vi "Magnetic_Force.vi"() -> ()   [LabVIEW 2022 SP3]
panel:
  out "Force (N/m)":dbl
  in  "Distance (m)":dbl
  in  "Current 2 (A)":dbl
  in  "Current 1 (A)":dbl
  # "Magnetic_Force:\n2 wires carrying a current will enact a \nmagnetic force upon each other. This force\nper unit length of wire will be calculated given\ninputs of current in each wire and the distance\nbetween said wires."
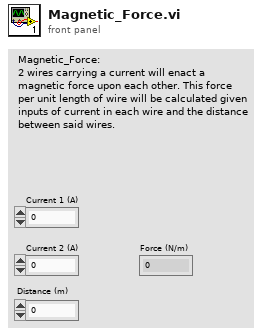
[diagram p1: front panel]
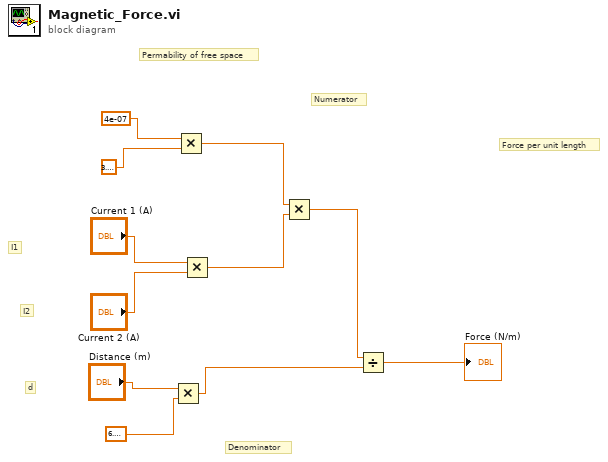
[diagram p0: block diagram]
diagram:
  # "Force per unit length"
  # "Denominator"
  # "Numerator"
  # "d"
  # "I2"
  # "I1"
  # "Permability of free space"
  n1 = Multiply(x="Distance (m)", y=6.283185307179586) -> (x*y=w2:dbl)
  n2 = Multiply(x=4e-07, y=3.141592653589793) -> (x*y=w7:dbl)
  n3 = Multiply(x="Current 1 (A)", y="Current 2 (A)") -> (x*y=w6:dbl)
  n4 = Multiply(x=w7, y=w6) -> (x*y=w3:dbl)
  n5 = Divide(x=w3, y=w2) -> (x/y=→"Force (N/m)":dbl)
